vi "FilterFromDTO.vi"(8 "error in (no error)":errorcluster, 11 "FilterDTO":T4={"mode"="Mirror", "levelMin"="INFO", "levelMax"="INFO", "tagPrefix"=""}) -> (0 "error out":errorcluster, 3 "Filter":T1={"mode"=enum."Mirror", "levelMin"=enum."INFO", "levelMax"=enum."INFO", "tagPrefix"=""})   [LabVIEW 2026, in "Lumberjack.lvlib"]
doc: "Maps a string FilterDTO back to the native Filter.\nParses mode to FilterMode and levelMin/levelMax to Severity (an unknown name raises a descriptive error); tagPrefix unchanged. Inverse of FilterDTOFromNative (SDD 4.2). No I/O.\nLumberjack.lvlib, community (friend of Tests.lvlib)."
uses:
  Lumberjack.lvlib
  TypeDefs/ConfigDTO/FilterDTO.ctl
  TypeDefs/Filter.ctl
  TypeDefs/FilterMode.ctl
  TypeDefs/Severity.ctl
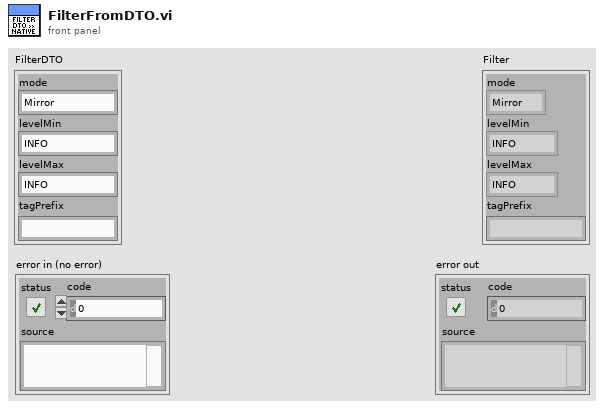
[diagram p1: front panel]
types:
  T1 = typedef "Lumberjack.lvlib/Filter.ctl" = cluster{"mode":T2, "levelMin":T3, "levelMax":T3, "tagPrefix":string}
  T2 = typedef "Lumberjack.lvlib/FilterMode.ctl" = enum16{"Mirror", "Routed"}
  T3 = typedef "Lumberjack.lvlib/Severity.ctl" = enum16{"OFF", "FATAL", "ERROR", "WARN", "INFO", "DEBUG", "TRACE", "ALL"}
  T4 = typedef "Lumberjack.lvlib/FilterDTO.ctl" = cluster{"mode":string, "levelMin":string, "levelMax":string, "tagPrefix":string}
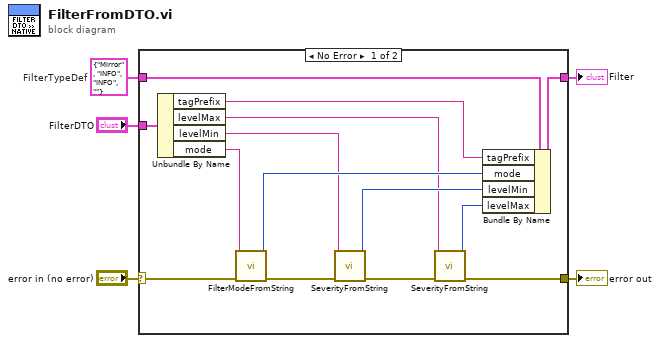
[diagram p0: block diagram]
diagram:
  w2 = T1 {"mode"=enum."Mirror", "levelMin"=enum."INFO", "levelMax"=enum."INFO", "tagPrefix"=""}  # FilterTypeDef
  n1 = case shown="No Error" "error in (no error)" {
    selector: "error in (no error)" -> [w19 w21]
    tunnel: [w16 w21] -> w4
    tunnel: "FilterDTO" -> [w11 _]
    tunnel: w2 -> [w6 w20]
    tunnel: [w15 w20] -> w1
    frame No Error {
      n2 = Unbundle By Name(w11) -> ("tagPrefix"=w10:string, "levelMax"=w7:string, "levelMin"=w8:string, "mode"=w9:string)
      n3 = call "FilterModeFromString.vi"("error in (no error)"=w19, "FilterModeString"=w9) -> ("error out"=w18:errorcluster, "FilterMode"=w12:T2)  [unwired: 8 in]
      n4 = call "SeverityFromString.vi"("error in (no error)"=w18, "SeverityString"=w8) -> ("error out"=w17:errorcluster, "Severity"=w13:T3)  [unwired: 8 in]
      n5 = call "SeverityFromString.vi"("error in (no error)"=w17, "SeverityString"=w7) -> ("error out"=w16:errorcluster, "Severity"=w14:T3)  [unwired: 8 in]
      n6 = Bundle By Name(cluster=w6, "tagPrefix"=w10, "mode"=w12, "levelMin"=w13, "levelMax"=w14) -> (w15:T1)
    }
    frame Error {
    }
  }
  "error out" <- w4
  "Filter" <- w1
